vi "SubVI_ProcessMaxOdtEntrySize.vi"(10 "Processor_KeyByte_IdentificationFieldType":u8, 11 "Current ODT Entry in":i32) -> (3 "Current ODT Entry out":i32)   [LabVIEW 2019, in "XCP_DaqDtoId.lvlib" / "DAQList.lvclass"]
uses:
  DAQList.lvclass
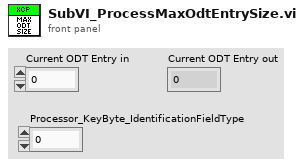
[diagram p1: front panel]
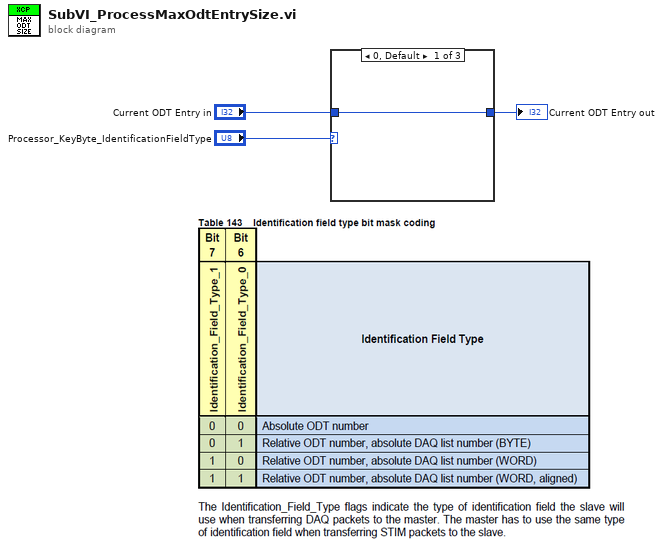
[diagram p0: block diagram]
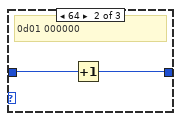
[diagram p2: hidden frame]
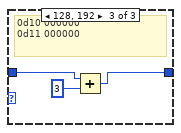
[diagram p3: hidden frame]
diagram:
  n1 = case shown="0, Default" "Processor_KeyByte_IdentificationFieldType" {
    tunnel: "Current ODT Entry in" -> [w4 w6 w9]
    tunnel: [w4 w5 w8] -> w1
    frame 0, Default {
    }
    frame 64 {
      # "0d01 000000"
      n2 = Increment(x=w6) -> (x+1=w5:i32)
    }
    frame 128, 192 {
      # "0d10 000000 \n0d11 000000"
      n3 = Add(x=w9, y=3) -> (x+y=w8:i32)
    }
  }
  "Current ODT Entry out" <- w1
